vi "InitiateGenerationRequest.vi"(8 "error in (no error)":errorcluster, 11 "ModuleID":i32) -> (0 "error out":errorcluster)   [LabVIEW 2014, in "FGenPlugins.lvlib" / "NISTFGenPluginsBase.lvclass"]
uses:
  NISTFGenPluginsBase.lvclass
  FGenModule/Protected/clEventType.ctl
  <vilib>/Utility/error.llb/Error Cluster From Error Code.vi
  <vilib>/ErrorRing/Error Ring.xnode
  FGenModule/FGenModule.lvlib
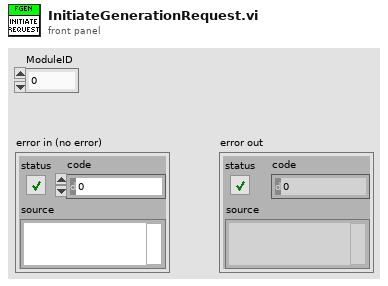
[diagram p1: front panel]
types:
  T1 = typedef "FGenModule.lvlib/clRequestEvents.ctl" = cluster{"StopRequest":refnum<user-event>, "PathToINI":refnum<user-event>, " LoadPlugin":refnum<user-event>, "OperateMode":refnum<user-event>, "OutputEnable":refnum<user-event>, "OutputMode":refnum<user-event>, "RefClkSource":refnum<user-event>, "ChannelName":refnum<user-event>, "Generation":refnum<user-event>, "AbortGeneration":refnum<user-event>, "Reset":refnum<user-event>, "Initialize":refnum<user-event>, "StdWaveform":refnum<user-event>, "ClrArbWfrm":refnum<user-event>, "CreateArbWfrm":refnum<user-event>, "ConfigArbWfrm":refnum<user-event>, "ConfigArbSRat":refnum<user-event>, "GetArbWfrm":refnum<user-event>, "ConfigTriigger":refnum<user-event>, "ShowPanel":refnum<user-event>, "ReadChannelParams":refnum<user-event>, "WriteChannelParams":refnum<user-event>, "ConfigDlg":refnum<user-event>}
  T2 = typedef "FGenModule.lvlib/clEventType.ctl" = cluster{"ModuleID":i32, "Data":variant}
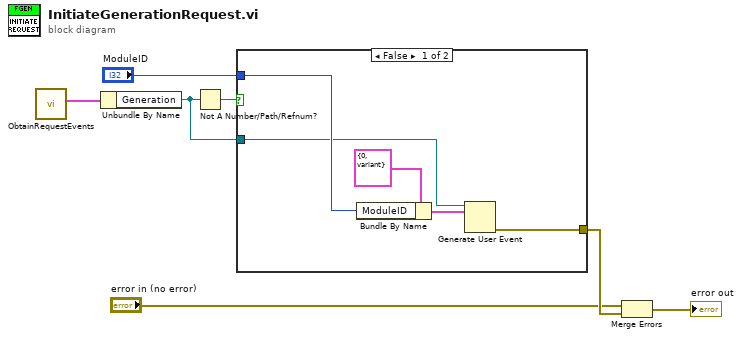
[diagram p0: block diagram]
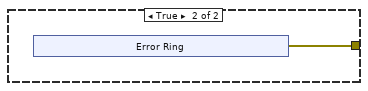
[diagram p2: hidden frame]
diagram:
  n1 = call "ObtainRequestEvents.vi"() -> ("clRequestEvents"=w7:T1)  [unwired: 10 in, 1 out]
  n2 = Unbundle By Name(w7) -> ("Generation"=w5:refnum<user-event>)
  n3 = Not A Number/Path/Refnum?(number/path/refnum=w5) -> (NaN/Path/Refnum?=w6:bool)
  n4 = case shown="False" w6 {
    tunnel: w5 -> [w9 _]
    tunnel: "ModuleID" -> [w11 _]
    tunnel: [w8 w13] -> w2
    frame False {
      n5 = Bundle By Name(cluster=T2 {"ModuleID"=0, "Data"=variant} ("clEventType"), "ModuleID"=w11) -> (w10:T2)
      n6 = Generate User Event(user event=w9, event data cluster=w10) -> (error out=w8:errorcluster)  [unwired: 2 in, 1 out]
    }
    frame True {
      n7 = xnode "Error Ring"() -> ("error out"=w13:errorcluster)
    }
  }
  n8 = Merge Errors("error in (no error)", w2) -> (→"error out":errorcluster)
